vi "AI RMS FGV.vi"(8 "error in":errorcluster, 10 "RMS value waveforms":waveform(dbl)[](array[waveform]), 11 "Enum":enum16{"Read", "Write"}(ring)) -> (0 "error out":errorcluster, 2 "RMS value waveforms":waveform(dbl)[](array[waveform]))   [LabVIEW 2022 SP3]
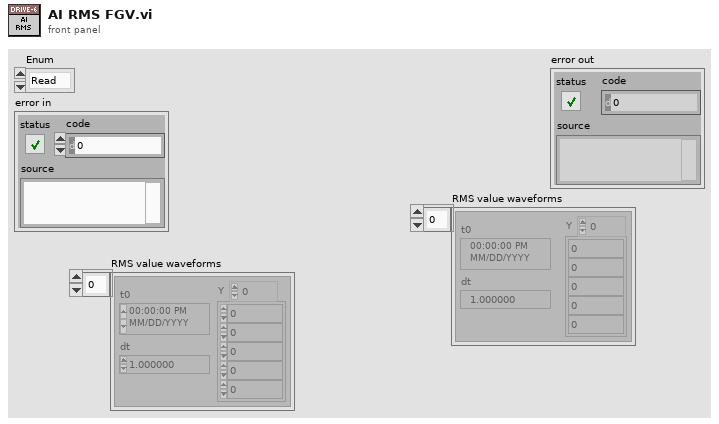
[diagram p1: front panel]
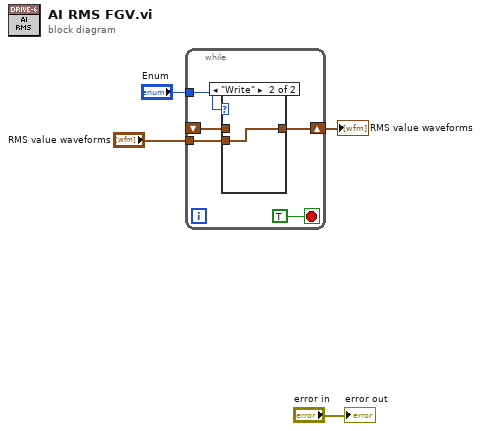
[diagram p0: block diagram]
diagram:
  n1 = while {
    tunnel: "Enum" -> [w9]
    tunnel: "RMS value waveforms" -> [w8]
    shift-right: [w7] -> w1
    shift-left: _ -> [w6]
    stop <- TRUE stop-if-true
    n2 = case shown="\"Write\"" w9 {
      tunnel: w8 -> [_ w11]
      tunnel: [w10 w11] -> w7
      tunnel: w6 -> [w10 _]
      frame "Read", Default {
      }
      frame "Write" {
      }
    }
  }
  "RMS value waveforms" <- w1
  "error out" <- "error in"
